vi "Initialize With Options.vi"(7 "option string":string, 8 "error in (no error)":errorcluster {"code" format="%.0x"}, 9 "reset device (Off)":bool, 10 "id query (Off)":bool, 11 "resource string":string caption="resource name") -> (0 "error out":errorcluster {"code" format="%.0x"}, 3 "instrument handle out":refnum<k15>)   [LabVIEW 2021, in "Keysight XSAnVMA.lvlib"]
doc: "Opens the I/O session to the instrument. Driver methods and properties that access the instrument are only accessible after Initialize is called. Initialize optionally performs a Reset and queries the instrument to validate the instrument model."
uses:
  <instrlib>/Keysight XSAnVMA/Keysight XSAnVMA.lvlib
  KtXSAnVMA_64.dll
panel:
  # "© Keysight Technologies 2018-2019"
  # "© 2000-2008 National Instruments.  All Rights Reserved."
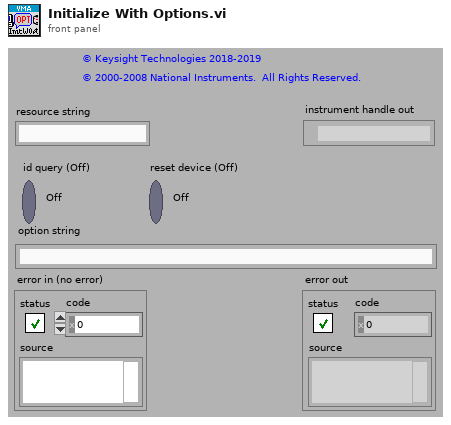
[diagram p1: front panel]
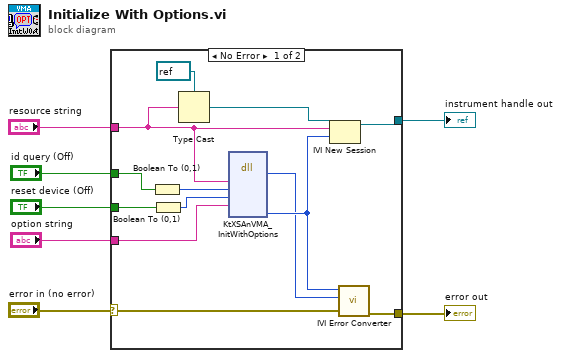
[diagram p0: block diagram]
diagram:
  n1 = case shown="No Error" "error in (no error)" {
    selector: "error in (no error)" -> [w13 w22]
    tunnel: [w14 w22] -> w6
    tunnel: "resource string" -> [w9 w21]
    tunnel: [w18 w21] -> w4
    tunnel: "option string" -> [w17 _]
    tunnel: "id query (Off)" -> [w16 _]
    tunnel: "reset device (Off)" -> [w15 _]
    frame No Error {
      n2 = Boolean To (0,1)(Boolean=w16) -> (0, 1=w20:i16)
      n3 = Boolean To (0,1)(Boolean=w15) -> (0, 1=w19:i16)
      n4 = Type Cast(type=refnum<k15> refnum ("instrument handle out"), x=w9) -> (*(type *) &x=w10:refnum<k15>)
      n5 = dll-call lib="KtXSAnVMA**.dll" fn="KtXSAnVMA_InitWithOptions" ("LabVIEW:Ivi_InitWithOptionsAndGetError")("resourceDescriptor"=w9, "idQuery"=w20, "reset"=w19, "optionString"=w17) -> ("return type"=w11:i32, "session"=w12:i32)  [unwired: 6 in, 4 out]
      n6 = IVI New Session(9:w12, 10:w9, 11:w10) -> (3:w18:refnum<k15>)
      n7 = call <instrlib>:"IVI Error Converter.vi"("error in (no error)"=w13, "IVI error code (0)"=w11, "instrument handle"=w12) -> ("error out"=w14:errorcluster)  [unwired: 7 in, 1 out]
    }
    frame Error {
    }
  }
  "error out" <- w6
  "instrument handle out" <- w4
